vi "LV8_6.vi"() -> ()   [LabVIEW 2016]
uses:
  <vilib>/imath/engines/lvmath2/RunTimeEngine/BuiltInFunctions/zeros/NIMS_V=zeros(I32,I32).vi
  <vilib>/imathl/engines/lvmath/Functions/Error Handling/Create Error.vi
  <vilib>/imath/engines/lvmath2/RunTimeEngine/IndexReplace/NIMS V(S)=S.vi
  <instcachedir>/0/NIMS V(S)=S_57E16554CB8B4B90AAB163894F717546.lvgen/NIMS V(S)=S_57E16554CB8B4B90AAB163894F717546_003.vi
  <instcachedir>/0/NIMS V(S)=S_57E16554CB8B4B90AAB163894F717546.lvgen/NIMS V(S)=S_57E16554CB8B4B90AAB163894F717546_000.vi
  <vilib>/imath/engines/lvmath2/RunTimeEngine/BuiltInFunctions/filter/NIMS_filter(GV,GV,GV,GV,Str).vi
  <instcachedir>/0/NIMS_filter(GV,GV,GV,GV,Str)_434E59EE96884CB3BC5141C85D3A0B2F.lvgen/NIMS_filter(GV,GV,GV,GV,Str)_434E59EE96884CB3BC5141C85D3A0B2F_000.vi
  <vilib>/imath/engines/lvmath2/RunTimeEngine/BuiltInFunctions/length/NIMS_length(GV).vi
  <instcachedir>/0/NIMS_length(GV)_08A3D13377FD4E4B96F5795FBF3698FA.lvgen/NIMS_length(GV)_08A3D13377FD4E4B96F5795FBF3698FA_002.vi
  <vilib>/imath/engines/lvmath2/RunTimeEngine/RangeToken/NIMS_Range.vi
  <instcachedir>/0/NIMS_Range_A7C094595B484CA7AF10685B02D808ED.lvgen/NIMS_Range_A7C094595B484CA7AF10685B02D808ED_001.vi
  <vilib>/imath/engines/lvmath2/RunTimeEngine/NodeEndStatement/NIMS_NodeEndStatement_Output.vi
  <instcachedir>/0/NIMS_NodeEndStatement_Output_53EC0D466D134D7ABD903AC30B43404B.lvgen/NIMS_NodeEndStatement_Output_53EC0D466D134D7ABD903AC30B43404B_005.vi
  <instcachedir>/0/NIMS_NodeEndStatement_Output_53EC0D466D134D7ABD903AC30B43404B.lvgen/NIMS_NodeEndStatement_Output_53EC0D466D134D7ABD903AC30B43404B_004.vi
  <vilib>/imath/engines/lvmath2/RunTimeEngine/ErrorHandling/NIMS_Finalize Error.vi
panel:
  out "Dereverbed Signal":cluster{"N":i32[], "Y":dbl[]}(graph)={"N"=[0, 1, 2, 3, 4, 5, 6, 7, 8, 9, 10, 11, 12, 13, 14, 15, 16, 17, 18, 19, 20, 21, 22, 23, 24, 25, 26, 27, 28, 29, 30], "Y"=[3.0000000000000053, -3.731628721304059e-14, 2.892335901431634e-15, 0.9999999999999957, 1.9761969838327786e-14, 6.2266616130988845e-15, 3.9999999999999547, 3.0295048154133086e-15, 9.103828801926284e-15, 1.000000000000002, 9.077862159895256e-15, 2.953535445326338e-14, 5.000000000000014, 1.9789725413943415e-14, 1.1629400030514747e-14, 8.99999999999999, 2.220446049250313e-14, 1.1546319456101628e-14, 8.331453935544327e-16, 1.1018963519404679e-14, -1.021405182655144e-14, 1.0127796322378522e-14, 1.1962056779141195e-14, -6.6058269965196814e-15, 5.773159728050814e-15, -4.269344209759107e-15, -7.127631818093505e-14, -3.0000775340857095e-14, -2.886579864025407e-15, -1.6764367671839864e-14, 5.014827712738342e-14]}
  in  "time delay":i32(slide)=1 scale=1.0..5.0
  in  "reflection coeff":dbl(slide)=0.6 scale=0.2..0.9
  out "Signal":cluster{"N":i32[], "X":i32[]}(graph)={"N"=[0, 1, 2, 3, 4, 5, 6, 7, 8, 9, 10, 11, 12, 13, 14, 15, 16, 17, 18, 19, 20, 21, 22, 23, 24, 25, 26, 27, 28, 29, 30], "X"=[3, 0, 0, 1, 0, 0, 4, 0, 0, 1, 0, 0, 5, 0, 0, 9, 0, 0, 0, 0, 0, 0, 0, 0, 0, 0, 0, 0, 0, 0, 0]}
  out "Reverbed Signal":cluster{"N":i32[], "Y":dbl[]}(graph)={"N"=[0, 1, 2, 3, 4, 5, 6, 7, 8, 9, 10, 11, 12, 13, 14, 15, 16, 17, 18, 19, 20, 21, 22, 23, 24, 25, 26, 27, 28, 29, 30], "Y"=[3.000000000000006, 1.7999999999999658, 1.0799999999999825, 1.647999999999986, 0.9888000000000108, 0.5932800000000124, 4.355967999999962, 2.61358079999998, 1.5681484799999967, 1.9408890880000003, 1.164533452800009, 0.6987200716800352, 5.419232043008035, 3.251539225804841, 1.950923535482916, 10.170554121289738, 6.102332472773865, 3.6613994836643293, 2.1968396901985985, 1.3181038141191692, 0.7908622884714915, 0.4745173730829046, 0.2847104238497551, 0.17082625430984644, 0.10249575258591401, 0.06149745155154307, 0.036898470930854466, 0.022139082558481887, 0.013283449535086912, 0.007970069721035231, 0.004782041832671225]}
  in  "stop":bool
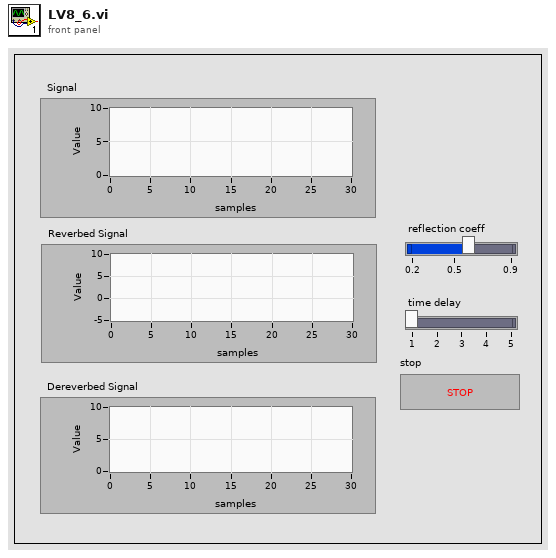
[diagram p1: front panel]
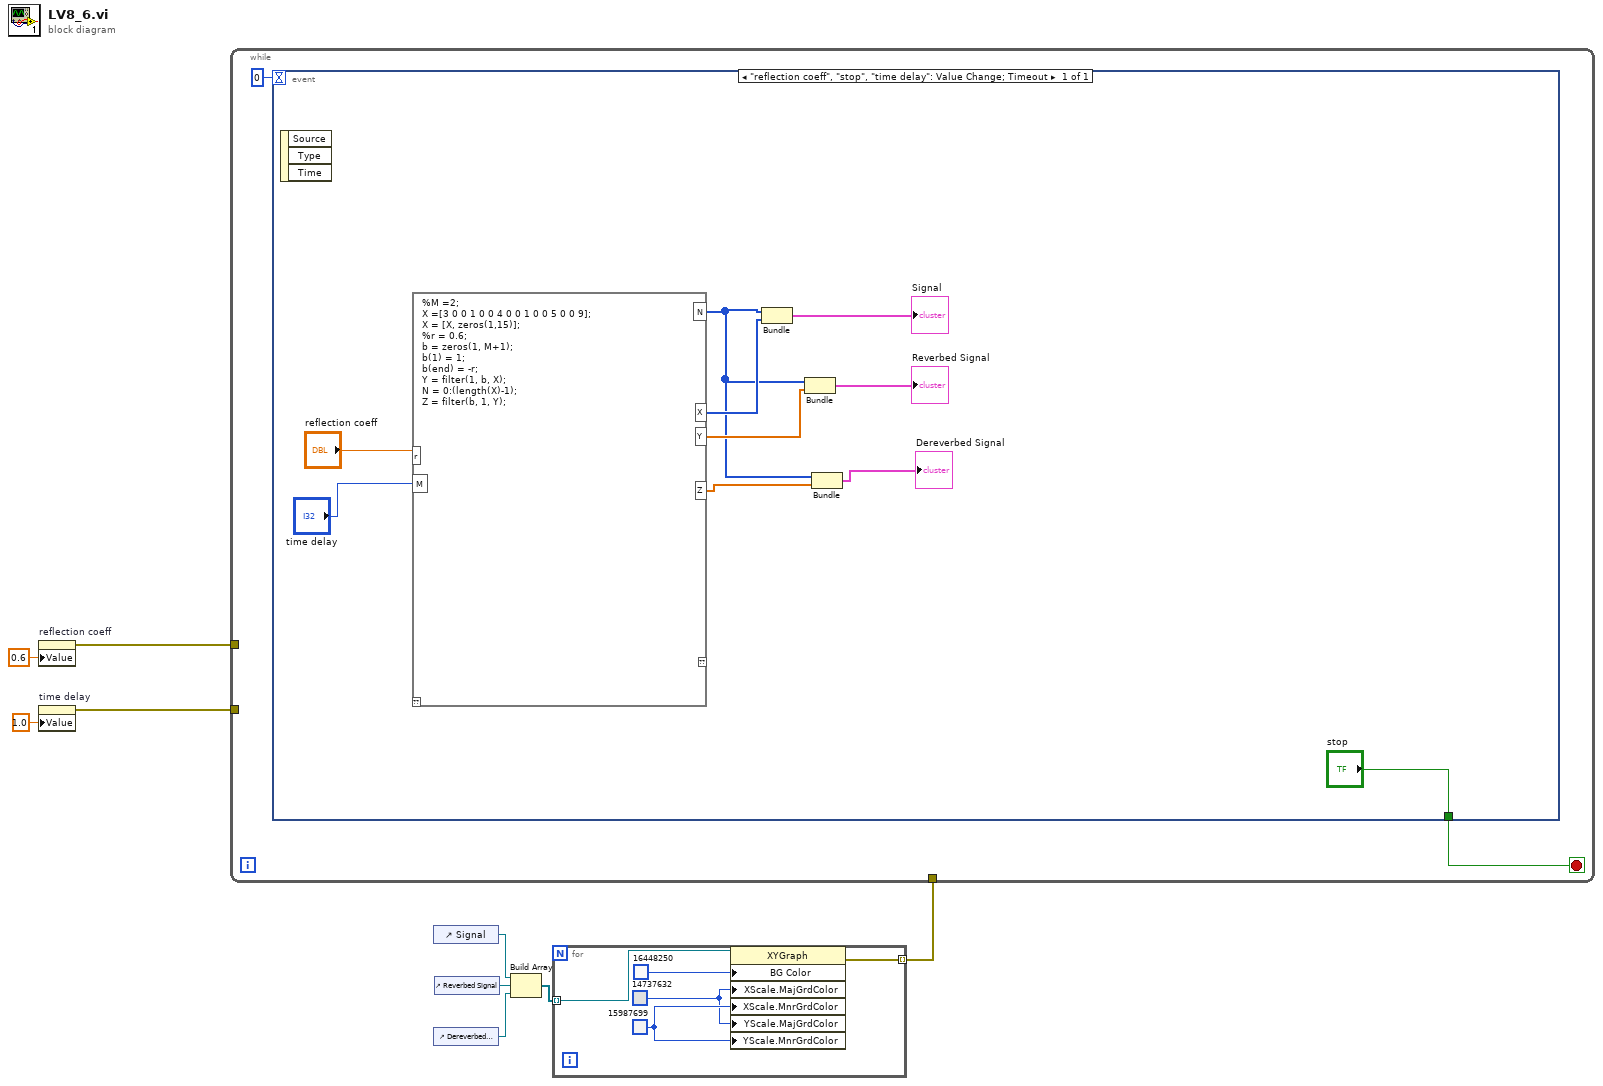
[diagram p0: block diagram]
diagram:
  n1 = property on="reflection coeff" class="Slide (strict)"("Value"=0.6 ("Interference level")) -> (error out=w9:errorcluster)  [unwired: 2 in, 1 out]
  n2 = property on="time delay" class="Slide (strict)"("Value"=1.0 ("notch frequency")) -> (error out=w7:errorcluster)  [unwired: 2 in, 1 out]
  n3 = control-ref of="Signal"() -> (w4:refnum<vi>)
  n4 = control-ref of="Dereverbed Signal"() -> (w2:refnum<vi>)
  n5 = control-ref of="Reverbed Signal"() -> (w3:refnum<vi>)
  n6 = Build Array(w4, w3, w2) -> (w5:refnum<vi>[])
  n7 = for {
    tunnel: w5 -> [w11] mode=indexing
    tunnel: [w10] -> w1 mode=indexing
    w13 = u32 15987699
    w12 = u32 14737632
    n8 = property class="XYGraph"(reference=w11, "BG Color"=u32 16448250, "XScale.MajGrdColor"=w12, "XScale.MnrGrdColor"=w13, "YScale.MajGrdColor"=w12, "YScale.MnrGrdColor"=w13) -> (error out=w10:errorcluster)  [unwired: 1 in, 1 out]
  }
  n9 = while {
    tunnel: w9 -> [_]
    tunnel: w7 -> [_]
    tunnel: w1 -> [_]
    stop <- w16 stop-if-true
    n10 = event shown="[0] \"reflection coeff\", \"stop\", \"time delay\": Value Change;  Timeout" {
      selector: _ -> [_]
      dyn-events: _ -> [_]
      timeout: 0 -> [_]
      tunnel: ["stop"] -> w16
      event "reflection coeff", "stop", "time delay": Value Change; Timeout {
        n11 = event-data() -> ()  [unwired: 1 in, 3 out]
        n12 = mathscript code="%M =2;\nX =[3 0 0 1 0 0 4 0 0 1 0 0 5 0 0 9];\nX = [X, zeros(1,15)];\n%r = 0.6;\nb = zeros(1, M+1);\nb(1) = 1;\nb(end) = -r;\nY = filter(1, b, X);\nN = 0:(length(X)-1);\nZ = filter(b, 1, Y);"("r"="reflection coeff", "M"="time delay") -> ("Y"=w23:dbl[], "X"=w24:i32[], "N"=w19:i32[], "Z"=w18:dbl[])  [unwired: 1 in, 1 out]
        n13 = Bundle("N"=w19, "X"=w24) -> (→"Signal":cluster{"N":i32[], "X":i32[]})  [unwired: 1 in]
        n14 = Bundle("N"=w19, "Y"=w23) -> (→"Reverbed Signal":cluster{"N":i32[], "Y":dbl[]})  [unwired: 1 in]
        n15 = Bundle("N"=w19, "Z"=w18) -> (→"Dereverbed Signal":cluster{"N":i32[], "Z":dbl[]})  [unwired: 1 in]
      }
    }
  }
